vi "DecodeRobot.vi"(1 "element":u8[](array[numeric]), 5 "error in (no error)":errorcluster) -> (14 "position":T1, 15 "element 2":u8[](array[numeric]), 19 "error out":errorcluster)   [LabVIEW 2023, in "Referee.lvclass"]
uses:
  Referee.lvclass
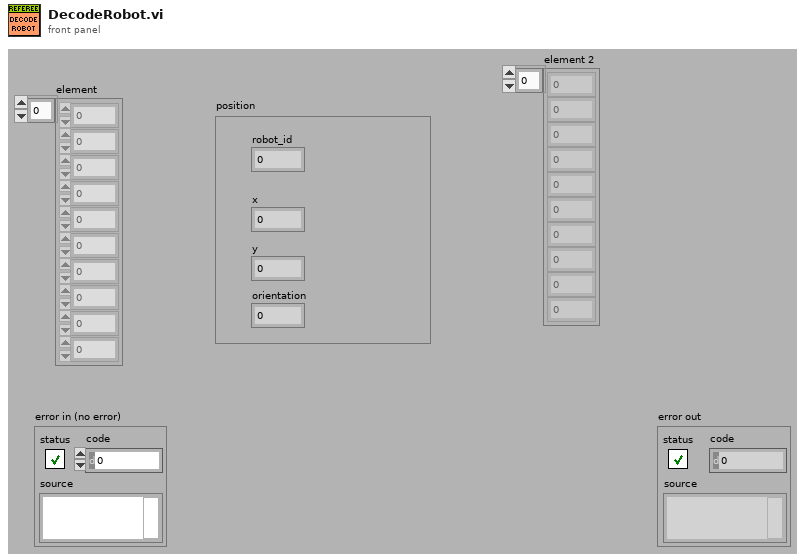
[diagram p1: front panel]
types:
  T1 = cluster{"robot_id":dbl, "x":dbl, "y":dbl, "orientation":dbl}
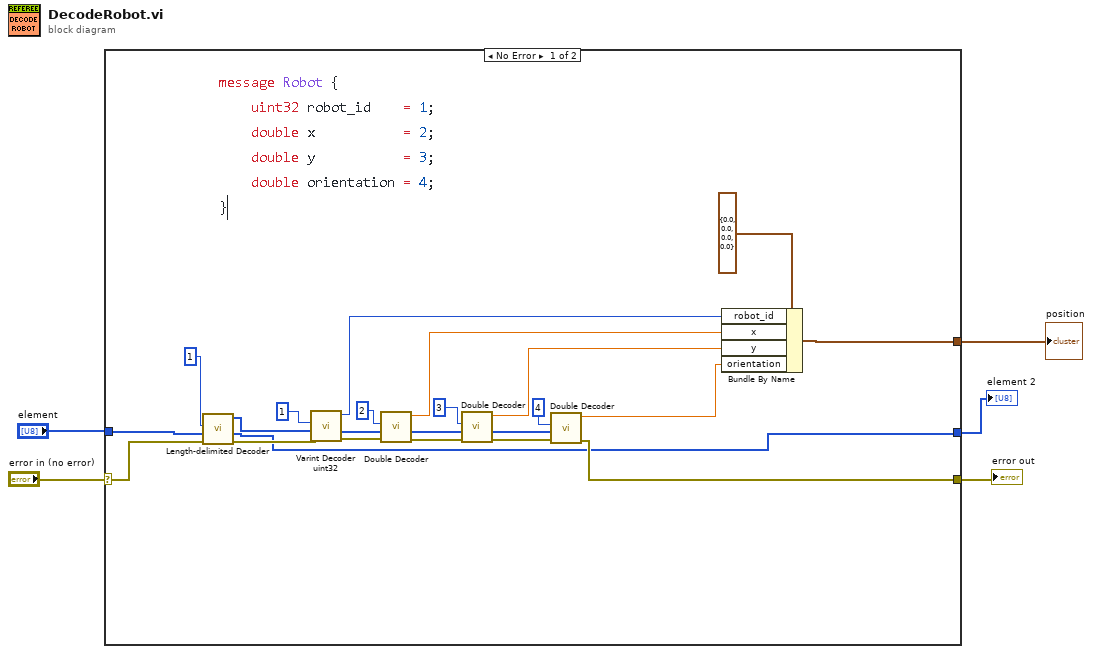
[diagram p0: block diagram]
diagram:
  n1 = case shown="No Error" "error in (no error)" {
    selector: "error in (no error)" -> [w9 w29]
    tunnel: [w16 w29] -> w4
    tunnel: "element" -> [w10 _]
    tunnel: [w18 _] -> w2
    tunnel: [w7 _] -> w1
    frame No Error {
      n2 = call "Length-delimited Decoder.vi"("error in (no error)"=w9, "Array"=w10, "Key"=1) -> ("error out"=w8:errorcluster, "array w/ subset deleted"=w7:u8[], "Length-delimited"=w6:u8[])  [unwired: 5 in, 1 out]
      n3 = call "Varint Decoder uint32.vi"("error in (no error)"=w8, "Array"=w6, "Key"=1) -> ("error out"=w26:errorcluster, "array w/ subset deleted"=w27:u8[], "Varint"=w15:u32)  [unwired: 5 in, 1 out]
      n4 = call "Double Decoder.vi"("error in (no error)"=w26, "Array"=w27, "Key"=2) -> ("error out"=w25:errorcluster, "array w/ subset deleted"=w24:u8[], "Double"=w14:dbl)  [unwired: 5 in, 1 out]
      n5 = call "Double Decoder.vi"("error in (no error)"=w25, "Array"=w24, "Key"=3) -> ("error out"=w23:errorcluster, "array w/ subset deleted"=w22:u8[], "Double"=w13:dbl)  [unwired: 5 in, 1 out]
      n6 = call "Double Decoder.vi"("error in (no error)"=w23, "Array"=w22, "Key"=4) -> ("error out"=w16:errorcluster, "Double"=w12:dbl)  [unwired: 5 in, 2 out]
      n7 = Bundle By Name(cluster=T1 {"robot_id"=0.0, "x"=0.0, "y"=0.0, "orientation"=0.0} ("position 2"), "robot_id"=w15, "x"=w14, "y"=w13, "orientation"=w12) -> (w18:T1)
    }
    frame Error {
    }
  }
  "error out" <- w4
  "element 2" <- w1
  "position" <- w2
